vi "HeaderuRayon.vi"(0 "Tester Software Ver":string, 2 "UUTHeader":string, 3 "UUT":string, 4 "S/N":string, 5 "VR":string, 6 "Oper.":string) -> (1 "HEADER1":string)   [LabVIEW 2017]
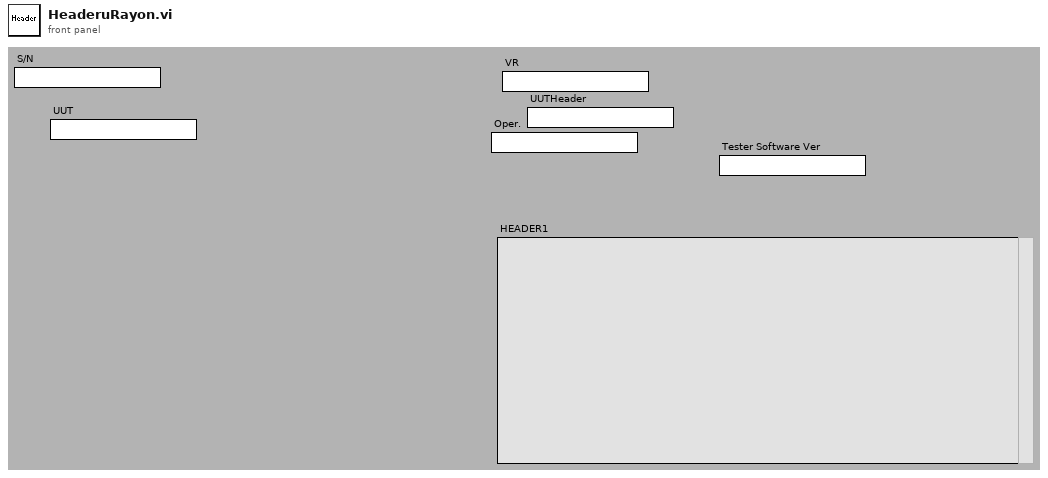
[diagram p1: front panel]
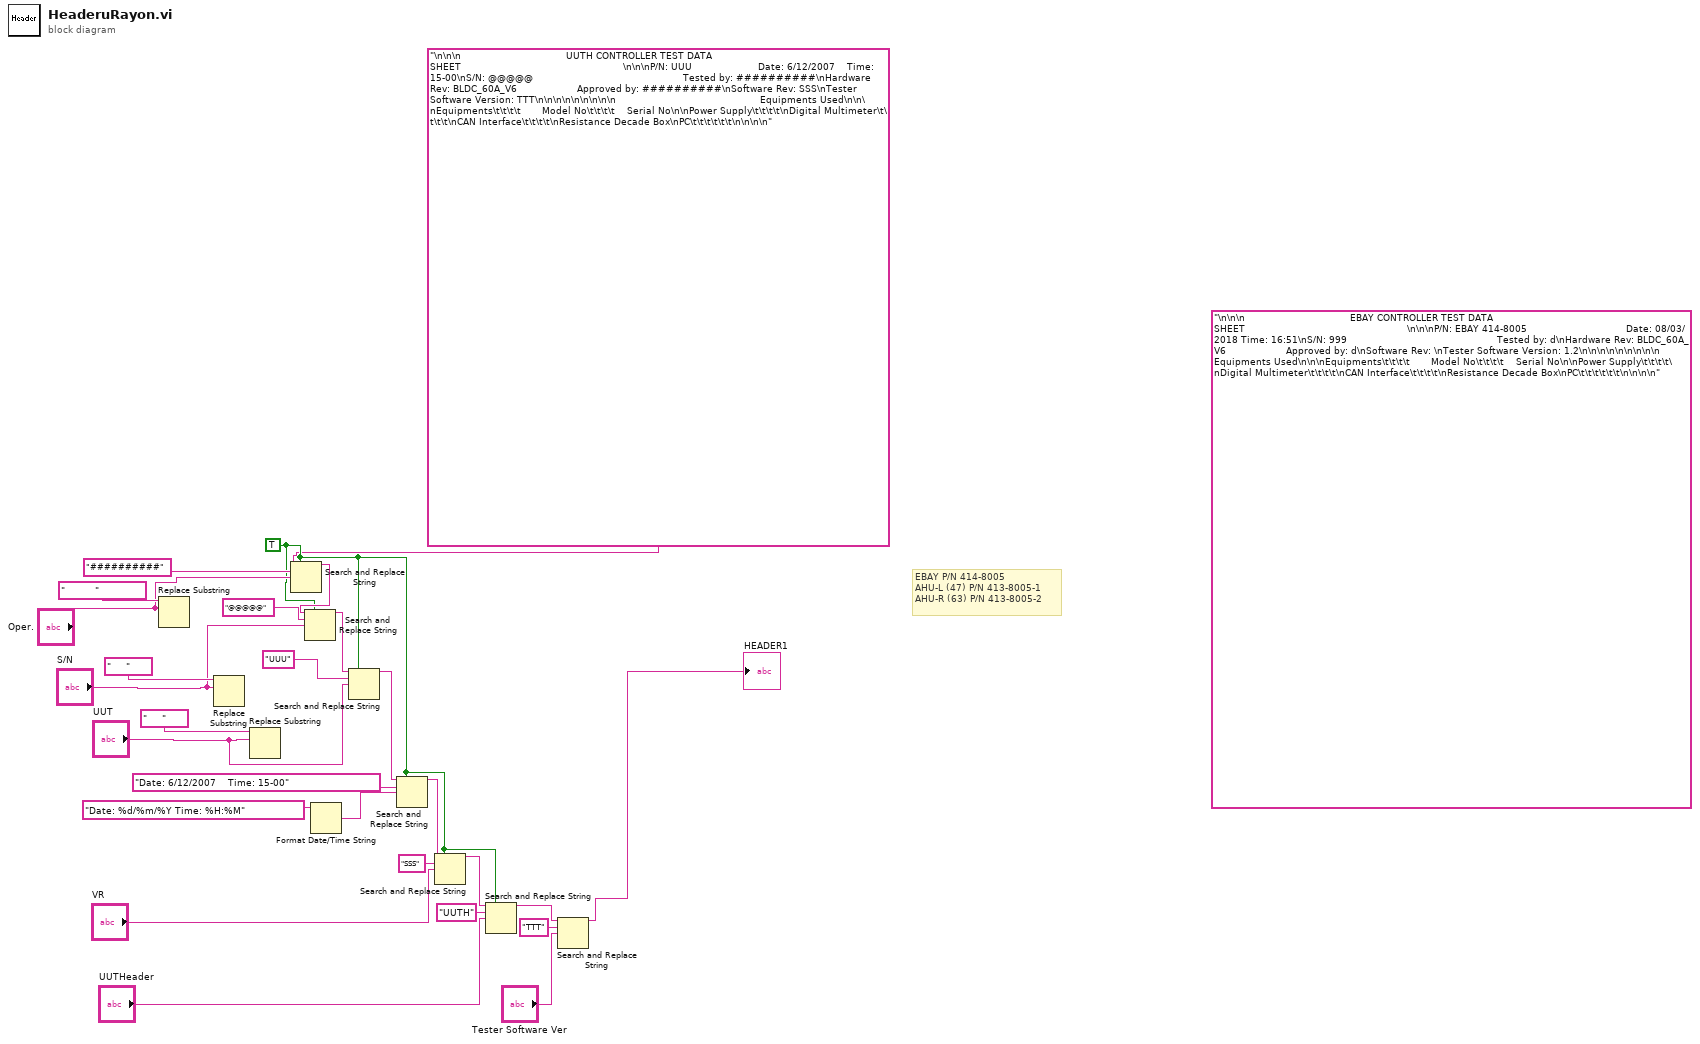
[diagram p0: block diagram]
diagram:
  (unwired) "\n\n\n                                   EBAY CONTROLLER TEST DATA SHEET                                                      \n\n\nP/N: EBAY 414-8005                                 Date: 08/03/2018 Time: 16:51\nS/N: 999                                                  Tested by: d\nHardware Rev: BLDC_60A_V6                    Approved by: d\nSoftware Rev: \nTester Software Version: 1.2\n\n\n\n\n\n\n\n\n                                                Equipments Used\n\n\nEquipments\t\t\t\t       Model No\t\t\t\t    Serial No\n\nPower Supply\t\t\t\t\nDigital Multimeter\t\t\t\t\nCAN Interface\t\t\t\t\nResistance Decade Box\nPC\t\t\t\t\t\t\n\n\n\n" ("HEADER1 2")
  w8 = TRUE ("replace all? (F)")
  # "EBAY P/N 414-8005\nAHU-L (47) P/N 413-8005-1\nAHU-R (63) P/N 413-8005-2"
  n1 = Replace Substring(4:"Oper.", 5:"          " ("source")) -> ()  [unwired: 2 in, 2 out]
  n2 = Replace Substring(4:"S/N", 5:"     " ("source")) -> ()  [unwired: 2 in, 2 out]
  n3 = Replace Substring(4:"UUT", 5:"     " ("source")) -> ()  [unwired: 2 in, 2 out]
  n4 = Search and Replace String(replace all?=w8, input string="\n\n\n                                   UUTH CONTROLLER TEST DATA SHEET                                                      \n\n\nP/N: UUU                      Date: 6/12/2007    Time: 15-00\nS/N: @@@@@                                                  Tested by: ##########\nHardware Rev: BLDC_60A_V6                    Approved by: ##########\nSoftware Rev: SSS\nTester Software Version: TTT\n\n\n\n\n\n\n\n\n                                                Equipments Used\n\n\nEquipments\t\t\t\t       Model No\t\t\t\t    Serial No\n\nPower Supply\t\t\t\t\nDigital Multimeter\t\t\t\t\nCAN Interface\t\t\t\t\nResistance Decade Box\nPC\t\t\t\t\t\t\n\n\n\n" ("result string"), search string="##########" ("source"), replace string="Oper.") -> (result string=w22:string)  [unwired: 4 in, 3 out]
  n5 = Search and Replace String(replace all?=w8, input string=w22, search string="@@@@@" ("source"), replace string="S/N") -> (result string=w17:string)  [unwired: 4 in, 3 out]
  n6 = Format Date/Time String(time format string (%c)="Date: %d/%m/%Y Time: %H:%M") -> (date/time string=w26:string)  [unwired: 2 in]
  n7 = Search and Replace String(replace all?=w8, input string=w17, search string="UUU" ("source"), replace string="UUT") -> (result string=w18:string)  [unwired: 4 in, 3 out]
  n8 = Search and Replace String(replace all?=w8, input string=w18, search string="Date: 6/12/2007    Time: 15-00" ("time format string (%c)"), replace string=w26) -> (result string=w12:string)  [unwired: 4 in, 3 out]
  n9 = Search and Replace String(replace all?=w8, input string=w12, search string="SSS", replace string="VR") -> (result string=w9:string)  [unwired: 4 in, 3 out]
  n10 = Search and Replace String(replace all?=w8, input string=w9, search string="UUTH", replace string="UUTHeader") -> (result string=w4:string)  [unwired: 4 in, 3 out]
  n11 = Search and Replace String(input string=w4, search string="TTT", replace string="Tester Software Ver") -> (result string=→"HEADER1":string)  [unwired: 5 in, 3 out]
